vi "Create&SaveNewVI.vi"(0 "Application ref in":refnum<vi>, 1 "VI name":string, 5 "VI path":path, 7 "Folder name":string, 9 "Project Path":path, 11 "error in (no error)":errorcluster) -> (4 "Application ref out":refnum<vi>, 6 "VI ref out":refnum<vi>, 15 "error out":errorcluster)   [LabVIEW 2016, in "ScriptSubVIs.lvlib"]
doc: "Creates a New VI as given in the template and saves it inside Tests folder in project location"
uses:
  ScriptSubVIs.lvlib
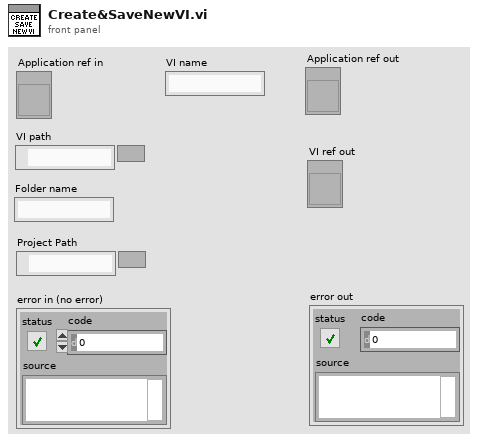
[diagram p1: front panel]
types:
  T1 = enum32{"invalid VI type", "Standard VI", "Control VI", "Global VI", "Polymorphic VI", "Configuration VI", "SubSystem", "Facade VI", "Method VI", "Statechart Diagram VI"}
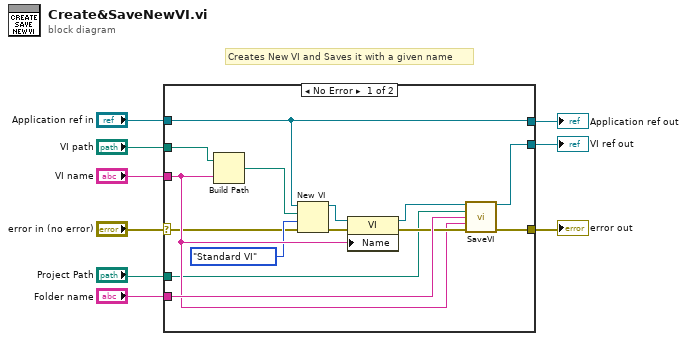
[diagram p0: block diagram]
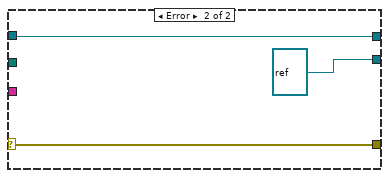
[diagram p2: hidden frame]
diagram:
  # "Creates New VI and Saves it with a given name"
  n1 = case shown="No Error" "error in (no error)" {
    selector: "error in (no error)" -> [w11 w26]
    tunnel: "Folder name" -> [w23 _]
    tunnel: [w22 refnum<vi> refnum ("VI out")] -> w8
    tunnel: [w21 w26] -> w7
    tunnel: "VI name" -> [w19 _]
    tunnel: "Project Path" -> [w18 _]
    tunnel: "Application ref in" -> [w10 w24]
    tunnel: "VI path" -> [w13 _]
    tunnel: [w10 w24] -> w1
    frame No Error {
      n2 = Build Path(base path=w13, name or relative path=w19) -> (appended path=w14:path)
      n3 = New VI(8:w11, 9:T1."Standard VI" ("vi type (standard vi)"), 10:w14, 11:w10) -> (0:w16:errorcluster, 3:w15:refnum<vi>)  [unwired: 3 in]
      n4 = property class="VI"(reference=w15, error in=w16, "Name"=w19) -> (reference out=w17:refnum<vi>, error out=w20:errorcluster)
      n5 = call "SaveVI.vi"("VI in"=w17, "Project Path"=w18, "Folder name"=w23, "VI name"=w19, "error in (no error)"=w20) -> ("VI out"=w22:refnum<vi>, "error out"=w21:errorcluster)  [unwired: 9 in]
    }
    frame Error {
    }
  }
  "VI ref out" <- w8
  "error out" <- w7
  "Application ref out" <- w1
